vi "FPGA_CounterEncoderSourceConvertionLVSourceTypeToFPGAType.vi"(8 "error in (no error)":errorcluster, 11 "DigitalSource":T1={"DevStatus"={"status"=FALSE, "code"=0, "source"=""}, "AnalogTriggerMode?"=FALSE, "DigitalMode"={"DIO Channel"=enum."DIO 1"}, "AnalogTriggerMode"={"AnalogTriggerIndex"=enum."Trig 0", "OutputType"=enum."InWindow"}}) -> (0 "error out":errorcluster, 3 "FPGASource":T5={"Channel"=2.0, "Module"=0.0, "AnalogTrigger"=FALSE})   [LabVIEW 2017]
uses:
  <vilib>/Rock Robotics/SystemInterfaces/CounterEncoderSourceConvertion/FPGA_CounterEncoderSourceConvertionLVSourceType.ctl
  <vilib>/Rock Robotics/SystemInterfaces/DIO/FPGA_DIODigitalSourceChannel.ctl
  <vilib>/Rock Robotics/SystemInterfaces/AnalogTrigger/FPGA_AnalogTriggerIndex.ctl
  <vilib>/Rock Robotics/SystemInterfaces/AnalogTrigger/FPGA_AnalogTriggerOutType.ctl
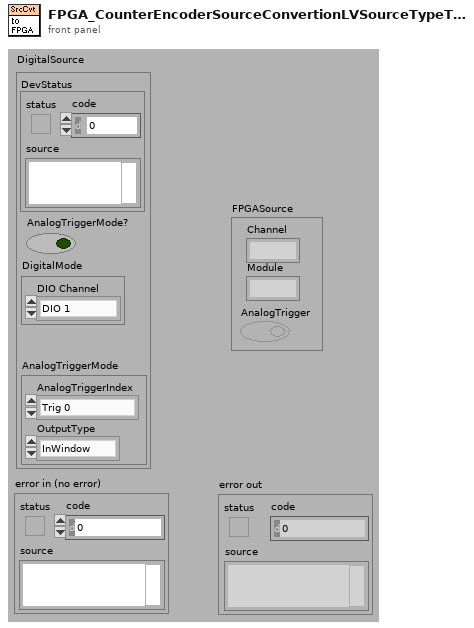
[diagram p1: front panel]
types:
  T1 = typedef "FPGA_CounterEncoderSourceConvertionLVSourceType.ctl" = cluster{"DevStatus":errorcluster, "AnalogTriggerMode?":bool, "DigitalMode":cluster{"DIO Channel":T2}, "AnalogTriggerMode":cluster{"AnalogTriggerIndex":T3, "OutputType":T4}}
  T2 = typedef "FPGA_DIODigitalSourceChannel.ctl" = enum8{"DIO 0", "DIO 1", "DIO 2", "DIO 3", "DIO 4", "DIO 5", "DIO 6", "DIO 7", "DIO 8", "DIO 9", "DIO MXP 0", "DIO MXP 1", "DIO MXP 2", "DIO MXP 3", "DIO MXP 4", "DIO MXP 5", "DIO MXP 6", "DIO MXP 7", "DIO MXP 8", "DIO MXP 9", "DIO MXP 10", "DIO MXP 11", "DIO MXP 12", "DIO MXP 13", "DIO MXP 14", "DIO MXP 15", "SPI Port CS1", "SPI Port CS2", "SPI Port CS3", "SPI Port MISO", "SPI Port MOSI", "Disabled"}
  T3 = typedef "FPGA_AnalogTriggerIndex.ctl" = enum8{"Trig 0", "Trig 1", "Trig 2", "Trig 3", "Trig 4", "Trig 5", "Trig 6", "Trig 7", "Invalid"}
  T4 = typedef "FPGA_AnalogTriggerOutType.ctl" = enum16{"InWindow", "TriggerState", "Rising", "Falling"}
  T5 = cluster{"Channel":fxp<+,4,4>, "Module":fxp<+,1,1>, "AnalogTrigger":bool}
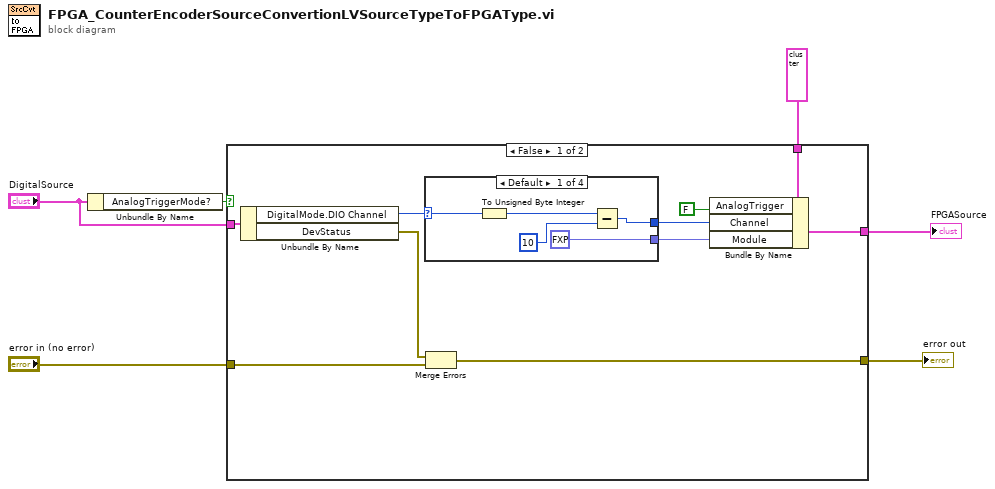
[diagram p0: block diagram]
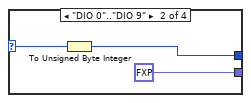
[diagram p2: hidden frame]
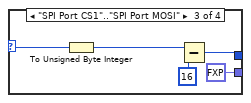
[diagram p3: hidden frame]
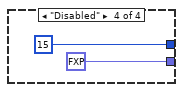
[diagram p4: hidden frame]
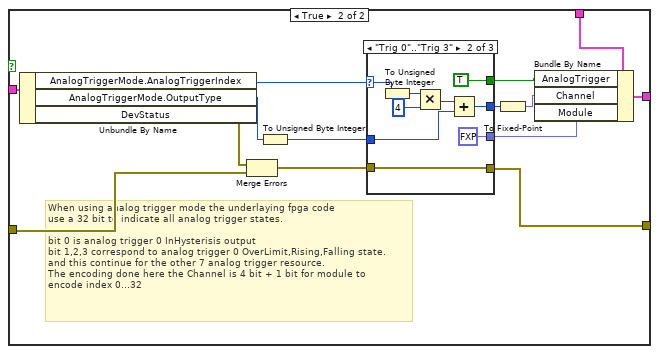
[diagram p5: hidden frame]
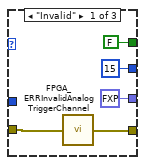
[diagram p6: hidden frame]
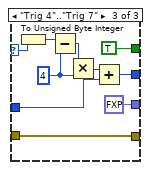
[diagram p7: hidden frame]
diagram:
  n1 = Unbundle By Name("DigitalSource") -> ("AnalogTriggerMode?"=w1:bool)
  n2 = case shown="False" w1 {
    tunnel: "DigitalSource" -> [w16 w43]
    tunnel: [w10 w37] -> w6
    tunnel: T5 {"Channel"=0.0, "Module"=0.0, "AnalogTrigger"=FALSE} ("FPGASource") -> [w15 w45]
    tunnel: [w14 w44] -> w4
    tunnel: "error in (no error)" -> [w12 w34]
    frame False {
      n3 = Unbundle By Name(w16) -> ("DigitalMode.DIO Channel"=w7:T2, "DevStatus"=w11:errorcluster)
      n4 = case shown="Default" w7 {
        selector: w7 -> [w20 w24 w26 _]
        tunnel: [w19 w22 w25 u8 15 ("unsigned 8bit integer")] -> w9
        tunnel: [fxp<+,1,1> 1.0 ("Module") fxp<+,1,1> 0.0 ("Module") fxp<+,1,1> 0.0 ("Module") fxp<+,1,1> 0.0 ("Module")] -> w8
        frame Default {
          n5 = To Unsigned Byte Integer(number=w20) -> (unsigned 8bit integer=w17:u8)
          n6 = Subtract(x=w17, y=u8 10) -> (x-y=w19:u8)
        }
        frame "DIO 0".."DIO 9" {
          n7 = To Unsigned Byte Integer(number=w24) -> (unsigned 8bit integer=w22:u8)
        }
        frame "SPI Port CS1".."SPI Port MOSI" {
          n8 = To Unsigned Byte Integer(number=w26) -> (unsigned 8bit integer=w27:u8)
          n9 = Subtract(x=w27, y=u8 16) -> (x-y=w25:u8)
        }
        frame "Disabled" {
        }
      }
      n10 = Merge Errors(w11, w12) -> (w10:errorcluster)
      n11 = Bundle By Name(cluster=w15, "AnalogTrigger"=FALSE, "Channel"=w9, "Module"=w8) -> (w14:T5)
    }
    frame True {
      # "When using analog trigger mode the underlaying fpga code\nuse a 32 bit to indicate all analog trigger states.\n\nbit 0 is analog trigger 0 InHysterisis output\nbit 1,2,3 correspond to analog trigger 0 OverLimit,Rising,Falling state.\nand this continue for the other 7 analog trigger resource.\nThe encoding done here the Channel is 4 bit + 1 bit for module to \nencode index 0...32"
      n12 = Unbundle By Name(w43) -> ("AnalogTriggerMode.AnalogTriggerIndex"=w36:T3, "AnalogTriggerMode.OutputType"=w42:T4, "DevStatus"=w35:errorcluster)
      n13 = Merge Errors(w35, w34) -> (w33:errorcluster)
      n14 = To Unsigned Byte Integer(number=w42) -> (unsigned 8bit integer=w41:u8)
      n15 = case shown="\"Trig 0\"..\"Trig 3\"" w36 {
        selector: w36 -> [_ w59 w69]
        tunnel: w41 -> [_ w55 w67]
        tunnel: [u8 15 w54 w66] -> w40
        tunnel: [fxp<+,1,1> 0.0 ("Module") fxp<+,1,1> 0.0 ("Module") fxp<+,1,1> 1.0 ("Module")] -> w39
        tunnel: [w47 w52 w61] -> w37
        tunnel: w33 -> [w48 w52 w61]
        tunnel: [FALSE ("AnalogTrigger") TRUE ("AnalogTrigger") TRUE ("AnalogTrigger")] -> w32
        frame "Invalid" {
          n16 = call <vilib>:"FPGA_ERRInvalidAnalogTriggerChannel.vi"("error in (no error)"=w48) -> ("error out"=w47:errorcluster)
        }
        frame "Trig 0".."Trig 3" {
          n17 = To Unsigned Byte Integer(number=w59) -> (unsigned 8bit integer=w58:u8)
          n18 = Multiply(x=w58, y=u8 4) -> (x*y=w56:u8)
          n19 = Add(x=w56, y=w55) -> (x+y=w54:u8)
        }
        frame "Trig 4".."Trig 7" {
          w64 = u8 4 ("y")
          n20 = To Unsigned Byte Integer(number=w69) -> (unsigned 8bit integer=w65:u8)
          n21 = Subtract(x=w65, y=w64) -> (x-y=w63:u8)
          n22 = Multiply(x=w63, y=w64) -> (x*y=w68:u8)
          n23 = Add(x=w68, y=w67) -> (x+y=w66:u8)
        }
      }
      n24 = To Fixed-Point(number=w40) -> (fixed-point=w38:fxp<+,4,4>)  [unwired: 1 out]
      n25 = Bundle By Name(cluster=w45, "AnalogTrigger"=w32, "Channel"=w38, "Module"=w39) -> (w44:T5)
    }
  }
  "FPGASource" <- w4
  "error out" <- w6
